vi "作业小朋友名字合并+排序.vi"() -> ()   [LabVIEW 2022 SP3]
uses:
  e1ac2560-31f0-4811-9484-5ad77935e292.vi
  <vilib>/Comparison/Less/Less Functor/Less Functor.lvclass
panel:
  out "数组":string[](array[string])
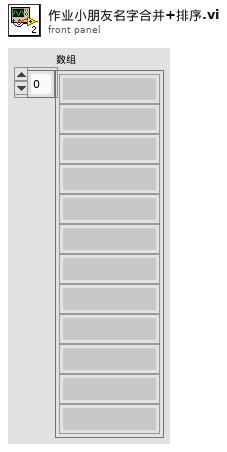
[diagram p1: front panel]
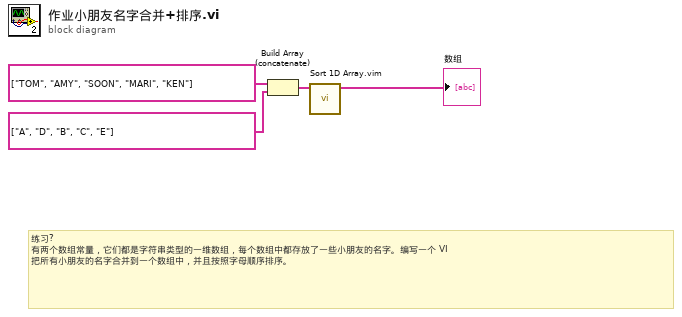
[diagram p0: block diagram]
diagram:
  # "练习?\n有两个数组常量，它们都是字符串类型的一维数组，每个数组中都存放了一些小朋友的名字。编写一个 VI 把所有小朋友的名字合并到一个数组中，并且按照字母顺序排序。"
  n1 = Build Array (concatenate)(string[] ["TOM", "AMY", "SOON", "MARI", "KEN"], string[] ["A", "D", "B", "C", "E"]) -> (w2:string[])
  n2 = call "Sort 1D Array.vim"("unsorted array"=w2) -> ("sorted array"=→"数组":string[])  [unwired: 10 in]
